vi "Example 1.vi"() -> ()   [LabVIEW 2020]
uses:
  lvFinanceFunctions/lvFinanceFunctionsHL.lvclass
panel:
  in  "Interval":T1(ring)
  in  "Period":T2(ring)
  in  "Ticker":string="MSFT"
  out "Market Data":cluster{timestamp[], dbl[]}[](graph)
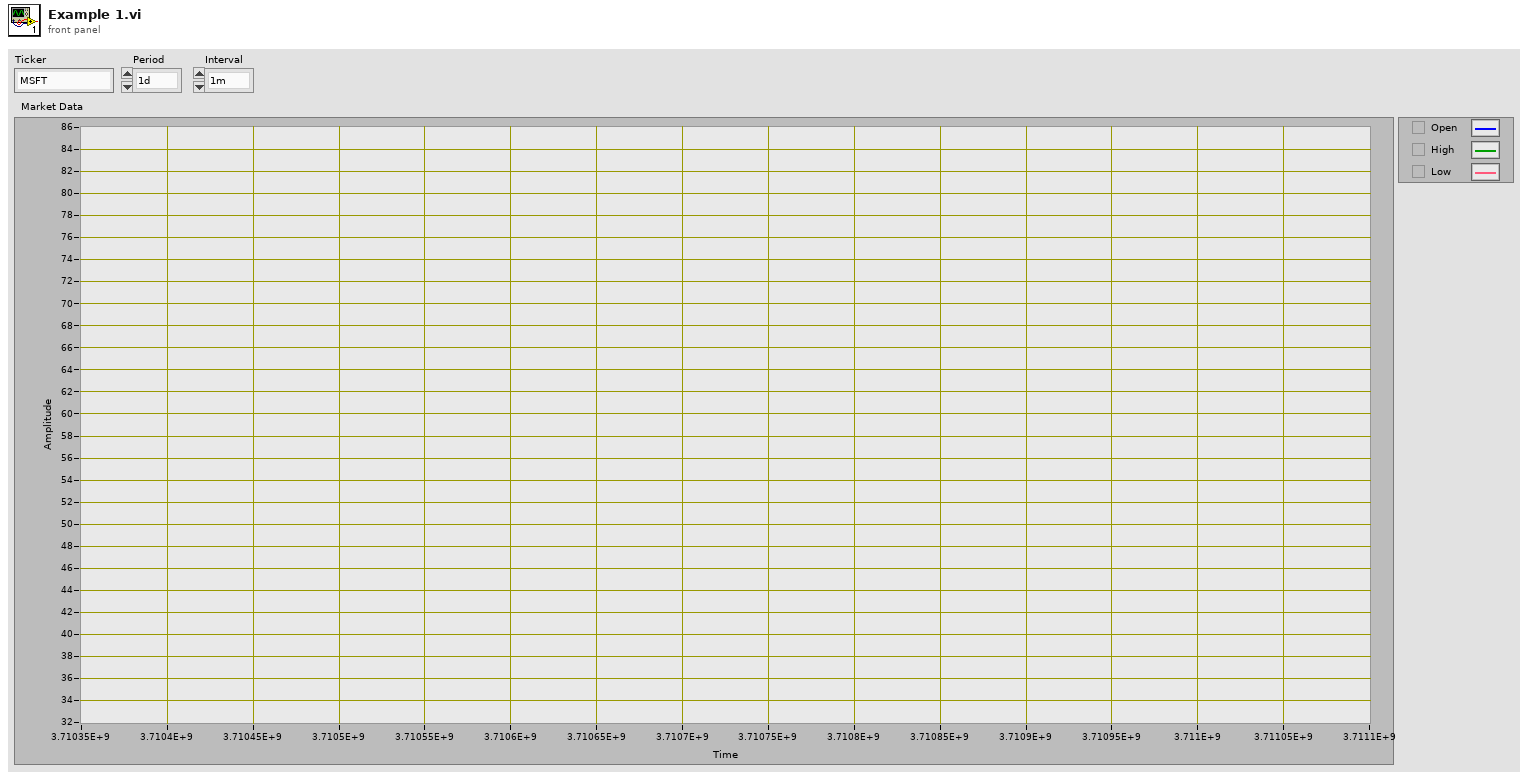
[diagram p1: front panel]
types:
  T1 = enum16{"1m", "2m", "5m", "15m", "30m", "60m", "90m", "1h", "1d", "5d", "1wk", "1mo", "3mo"}
  T2 = enum16{"1d", "5d", "1mo", "3mo", "6mo", "1y", "2y", "5y", "10y", "ytd", "max"}
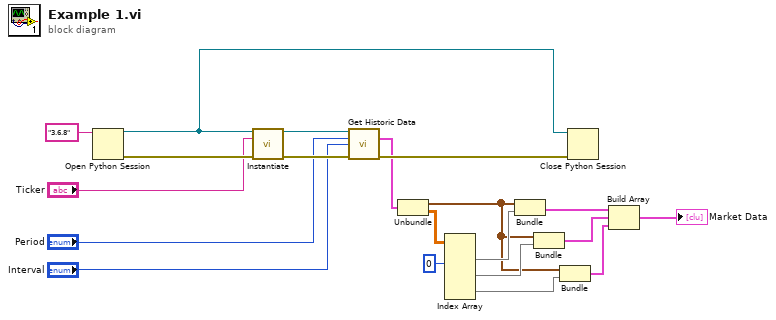
[diagram p0: block diagram]
diagram:
  n1 = Open Python Session(python version="3.6.8" ("Python version")) -> (session out=w18:refnum<k35>, error out=w19:errorcluster)  [unwired: 2 in]
  n2 = call "Instantiate.vi"("py session"=w18, "Ticker"="Ticker", "error in"=w19) -> ("lvFinanceFunctionsHL out"=w17:refnum<class "lvFinanceFunctionsHL.lvclass">, "error out"=w16:errorcluster)  [unwired: 11 in]
  n3 = call-dynamic "Get Historic Data.vi"("lvFinanceFunctionsHL in"=w17, "Period"="Period", "Interval"="Interval", "error in (no error)"=w16) -> ("Historic Data"=w11:cluster{timestamp[], dbl[][]}, "error out"=w15:errorcluster)  [unwired: 9 in, 1 out]
  n4 = Unbundle(w11) -> (w6:timestamp[], w10:dbl[][])
  n5 = Index Array(array=w10, index (col) #1=0 ("disabled index (col)")) -> (element #1=w8:dbl[], element #2=w7:dbl[], element #3=w5:dbl[])  [unwired: 5 in]
  n6 = Bundle(w6, w8) -> (w4:cluster{timestamp[], dbl[]})  [unwired: 1 in]
  n7 = Bundle(w6, w7) -> (w2:cluster{timestamp[], dbl[]})  [unwired: 1 in]
  n8 = Bundle(w6, w5) -> (w3:cluster{timestamp[], dbl[]})  [unwired: 1 in]
  n9 = Close Python Session(session in=w18, error in=w15) -> ()  [unwired: 1 out]
  n10 = Build Array(w4, w2, w3) -> (→"Market Data":cluster{timestamp[], dbl[]}[])
